vi "Set Channel.vi"(8 "error in (no error)":errorcluster, 10 "Channel":refnum<class "CIFChannels.lvclass">, 11 "CIFCorePlugin in":refnum<class "CIFCorePlugin.lvclass">) -> (0 "error out":errorcluster, 3 "CIFCorePlugin out":refnum<class "CIFCorePlugin.lvclass">)   [LabVIEW 2021, in "CIFCorePlugin.lvclass"]
uses:
  CIFCorePlugin.lvclass
  CIFCorePlugin.lvclass/CIFCorePlugin.ctl
  CIFUtilities/CIFChannelMng/CIFChannelMng.lvclass
  CIFUtilities/CIFChannels/CIFChannels.lvclass
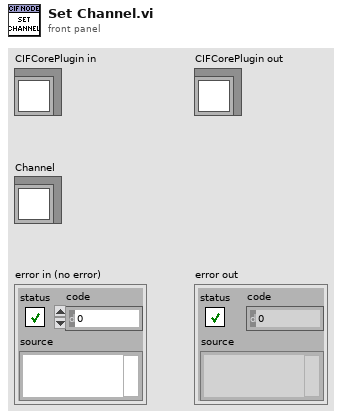
[diagram p1: front panel]
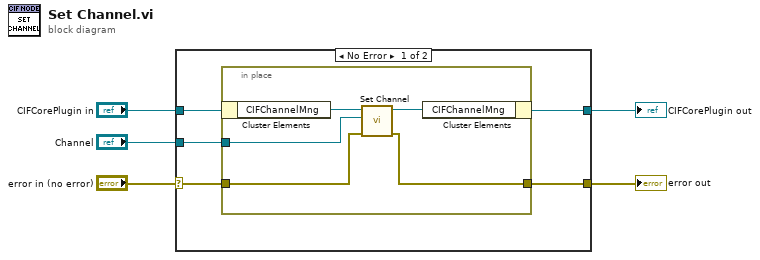
[diagram p0: block diagram]
diagram:
  n1 = case shown="No Error" "error in (no error)" {
    selector: "error in (no error)" -> [w7 w17]
    tunnel: [w6 w17] -> w4
    tunnel: [w9 w16] -> w2
    tunnel: "CIFCorePlugin in" -> [w10 w16]
    tunnel: "Channel" -> [w8 _]
    frame No Error {
      n2 = in-place {
        in-place-border: w8 -> [w11]
        in-place-border: w7 -> [w13]
        in-place-border: [w12] -> w6
        n3 = in-place-cluster #1(w10) -> ("CIFChannelMng"=w15:refnum<class "CIFChannelMng.lvclass">)
        n4 = call "Set Channel.vi"("error in (no error)"=w13, "Channel"=w11, "CIFChannelMng in"=w15) -> ("error out"=w12:errorcluster, "CIFChannelMng out"=w14:refnum<class "CIFChannelMng.lvclass">)  [unwired: 7 in]
        n5 = in-place-cluster #1("CIFChannelMng"=w14) -> (w9:refnum<class "CIFCorePlugin.lvclass">)
      }
    }
    frame Error {
    }
  }
  "error out" <- w4
  "CIFCorePlugin out" <- w2
